vi "GT_Read_Config.vi"(4 "error in (no error)":errorcluster, 7 "Config Refnum":T1) -> (0 "error out":errorcluster, 2 "All Found?":bool, 3 "refnum out":T1)   [LabVIEW 2015]
uses:
  <vilib>/Utility/config.llb/Config Data RefNum.ctl
  <vilib>/Utility/config.llb/Read Key (I32).vi
  Systems/Grating_Translation/GSP_GT_Global.vi
  <vilib>/Utility/config.llb/NI_LVConfig.lvlib
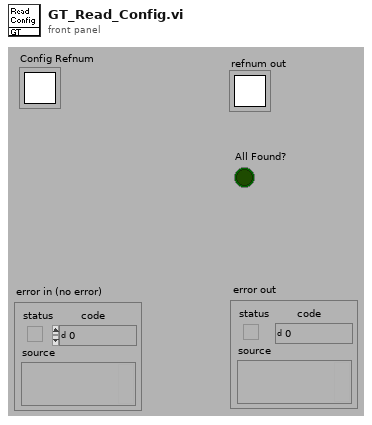
[diagram p1: front panel]
types:
  T1 = typedef "NI_LVConfig.lvlib/Config Data RefNum.ctl" = refnum<k1>
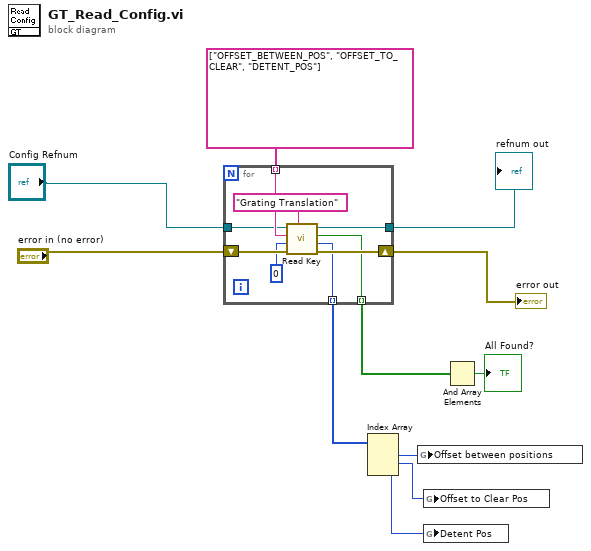
[diagram p0: block diagram]
diagram:
  n1 = for {
    shift-right: [w18] -> w7
    shift-left: "error in (no error)" -> [w20]
    tunnel: [w17] -> w8
    tunnel: string[] ["OFFSET_BETWEEN_POS", "OFFSET_TO_CLEAR", "DETENT_POS"] -> [w16] mode=indexing
    tunnel: "Config Refnum" -> [w15]
    tunnel: [w13] -> w5 mode=indexing
    tunnel: [w12] -> w6 mode=indexing
    n2 = call-poly <vilib>:"Read Key.vi"("section"="Grating Translation", "error in (no error)"=w20, "default value"=0, "key"=w16, "refnum"=w15) -> ("error out"=w18:errorcluster, "value"=w13:i32, "found?"=w12:bool, "refnum out"=w17:T1)  [unwired: 3 in]
  }
  "error out" <- w7
  "refnum out" <- w8
  n3 = Index Array(array=w5) -> (element #1=w2:i32, element #2=w3:i32, element #3=w1:i32)  [unwired: 3 in]
  n4 = global write "GSP_GT_Global.vi" "Offset between positions"(w2) -> ()
  n5 = global write "GSP_GT_Global.vi" "Offset to Clear Pos"(w3) -> ()
  n6 = global write "GSP_GT_Global.vi" "Detent Pos"(w1) -> ()
  n7 = And Array Elements(Boolean array=w6) -> (logical AND=→"All Found?":bool)
